vi "Convert HeadSaveOptions to U32.vi"(2 "HeadSaveOptions in":T1) -> (16 "HeadSaveOptions out":u32)   [LabVIEW 2013, in "VRI.lvlib"]
uses:
  VRI.lvlib
  _Type Defs/PhFile HeadSaveOptions.ctl
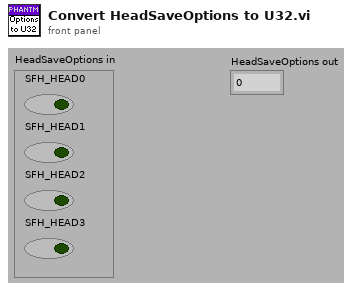
[diagram p1: front panel]
types:
  T1 = typedef "VRI.lvlib/PhFile HeadSaveOptions.ctl" = cluster{"SFH_HEAD0":bool, "SFH_HEAD1":bool, "SFH_HEAD2":bool, "SFH_HEAD3":bool}
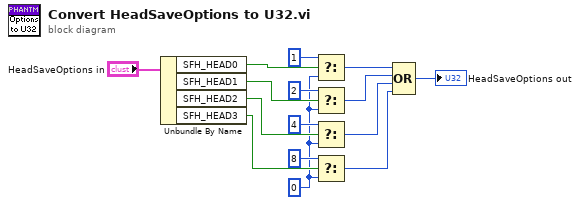
[diagram p0: block diagram]
diagram:
  w5 = u32 0 ("f")
  n1 = Unbundle By Name("HeadSaveOptions in") -> ("SFH_HEAD0"=w14:bool, "SFH_HEAD1"=w11:bool, "SFH_HEAD2"=w12:bool, "SFH_HEAD3"=w13:bool)
  n2 = Select(t=u32 1, s=w14, f=w5) -> (s? t:f=w6:u32)
  n3 = Select(t=u32 2, s=w11, f=w5) -> (s? t:f=w2:u32)
  n4 = Select(t=u32 4, s=w12, f=w5) -> (s? t:f=w3:u32)
  n5 = Select(t=u32 8, s=w13, f=w5) -> (s? t:f=w4:u32)
  n6 = Compound Arithmetic op=OR(w6, w2, w3, w4) -> (→"HeadSaveOptions out":u32)
